vi "Format JSON Object.vi"(8 "error in (no error)":errorcluster, 9 "Pretty Print?":bool, 10 "JSON elements":string[](array[string]), 11 "Names":string[](array[string])) -> (0 "error out":errorcluster, 3 "JSON Object Text out":string)   [LabVIEW 2020, in "Library Commun.lvlib" / "JSON support.lvlib"]
uses:
  support/JSON support.lvlib
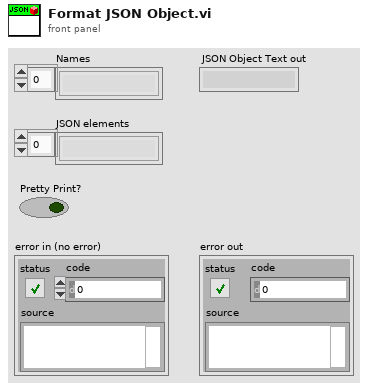
[diagram p1: front panel]
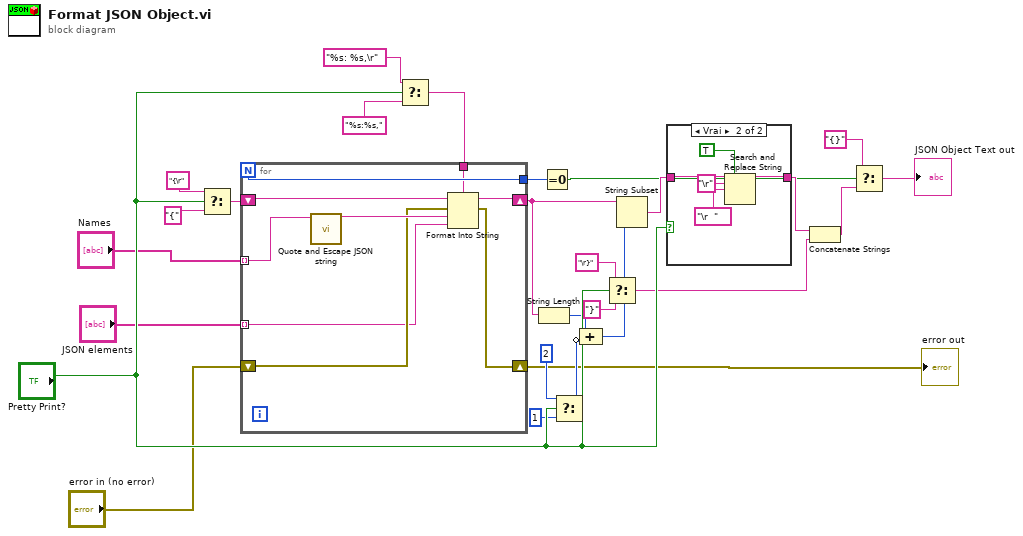
[diagram p0: block diagram]
diagram:
  n1 = Select(t="{\r", s="Pretty Print?", f="{") -> (s? t:f=w10:string)
  n2 = Select(t="%s: %s,\r" ("format string"), s="Pretty Print?", f="%s:%s," ("format string")) -> (s? t:f=w21:string)
  n3 = for {
    N -> [w33]
    tunnel: "Names" -> [w31] mode=indexing
    tunnel: "JSON elements" -> [w28] mode=indexing
    shift-right: [w34] -> w8
    shift-left: w10 -> [w36]
    shift-right: [w35] -> w2
    shift-left: "error in (no error)" -> [w29]
    tunnel: [w33] -> w3
    tunnel: w21 -> [w32]
    n4 = call "Quote and Escape JSON string.vi"("Plain Text"=w31) -> ("<JSON>"=w30:string)  [unwired: 10 in]
    n5 = Format Into String(format string=w32, initial string=w36, error in=w29, w30, w28) -> (resulting string=w34:string, error out=w35:errorcluster)
  }
  "error out" <- w2
  n6 = String Length(string=w8) -> (length=w7:i32)
  n7 = Equal To 0?(x=w3) -> (x = 0?=w4:bool)
  n8 = Select(t=2, s="Pretty Print?", f=1) -> (s? t:f=w24:i32)
  n9 = Compound Arithmetic op=ADD(w7, invert w24) -> (w9:i32)
  n10 = Select(t="\r}" ("substring (\"\")"), s="Pretty Print?", f="}" ("substring (\"\")")) -> (s? t:f=w13:string)
  n11 = String Subset(string=w8, length (rest)=w9) -> (substring=w15:string)  [unwired: 1 in]
  n12 = case shown="Vrai" "Pretty Print?" {
    tunnel: w15 -> [w37 w42]
    tunnel: [w37 w41] -> w16
    frame False {
    }
    frame True {
      n13 = Search and Replace String(replace all?=TRUE ("replace all? (F)"), input string=w42, search string="\r", replace string="\r  " ("search string")) -> (result string=w41:string)  [unwired: 4 in, 3 out]
    }
  }
  n14 = Concatenate Strings(w16, w13) -> (w17:string)
  n15 = Select(t="{}", s=w4, f=w17) -> (s? t:f=→"JSON Object Text out":string)
